vi "DialogUsingEvents 1.vi"(10 "Strings []":string[](array[string])) -> (1 "element":string, 2 "Numeric":i32 caption="Выбери файл для редактирования", 3 "Cancelled?":bool)   [LabVIEW 2010]
doc: "Use this template to create a dialog box with event handling."
panel:
  in  "Ring":u16(ring) caption="Выбери файл для редактирования" items=["shed.txt", "err.log", "5.ini"]
  in  "Cancel":bool
  in  "OK":bool
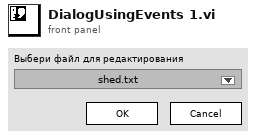
[diagram p1: front panel]
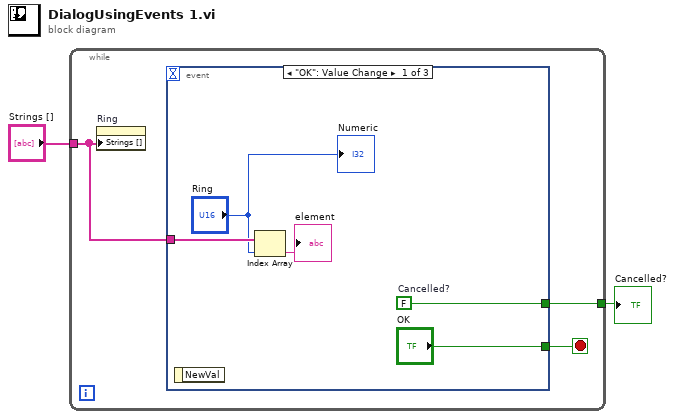
[diagram p0: block diagram]
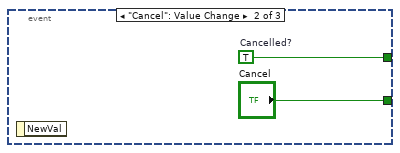
[diagram p2: hidden frame]
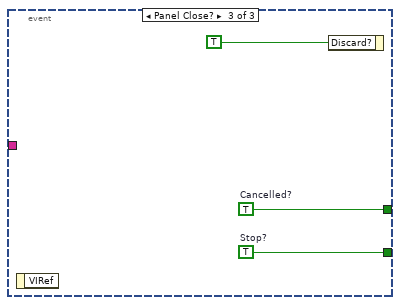
[diagram p3: hidden frame]
diagram:
  n1 = while {
    tunnel: [w4] -> w2
    tunnel: "Strings []" -> [w3]
    stop <- w5 stop-if-true
    n2 = property on="Ring" class="Ring (strict)"("Strings []"=w3) -> ()  [unwired: 2 in, 2 out]
    n3 = event shown="[0] \"OK\": Value Change" {
      selector: _ -> [_ _ _]
      dyn-events: _ -> [_ _ _]
      timeout: _ -> [_ _ _]
      tunnel: ["OK" "Cancel" w14] -> w5
      tunnel: [w10 w12 w13] -> w4
      tunnel: w3 -> [w8 _ _]
      event "OK": Value Change {
        w10 = FALSE  # Cancelled?
        n4 = event-data() -> ()  [unwired: 1 in, 1 out]
        n5 = Index Array(array=w8, index="Ring") -> (element=→"element":string)
        "Numeric" <- "Ring"
      }
      event "Cancel": Value Change {
        w12 = TRUE  # Cancelled?
        n6 = event-data() -> ()  [unwired: 1 in, 1 out]
      }
      event Panel Close? {
        w13 = TRUE  # Cancelled?
        w14 = TRUE  # Stop?
        n7 = event-data() -> ()  [unwired: 1 in, 1 out]
        n8 = event-data("Discard?"=TRUE) -> ()  [unwired: 1 in, 1 out]
      }
    }
  }
  "Cancelled?" <- w2
